vi "SetBuildVersionCaller.vi"(11 "Command line arguments \nfor the VI":string[](array[string])) -> (2 "Output or error information to include in \nthe CLI for LabVIEW console or log file.":string, 3 "CLI for LabVIEW exit code that the VI returns":i32)   [LabVIEW 2020]
doc: "Calls SetBuildVersion.vi to set the version of the build specification."
uses:
  <vilib>/AppBuilder/AB_API_Simple/Build Specification Version.ctl
  <vilib>/AppBuilder/AB_API_Simple/NI_App_Builder_API.lvlib
panel:
  out "error out":errorcluster
  in  "error in (no error)":errorcluster
  out "Set Version":T1
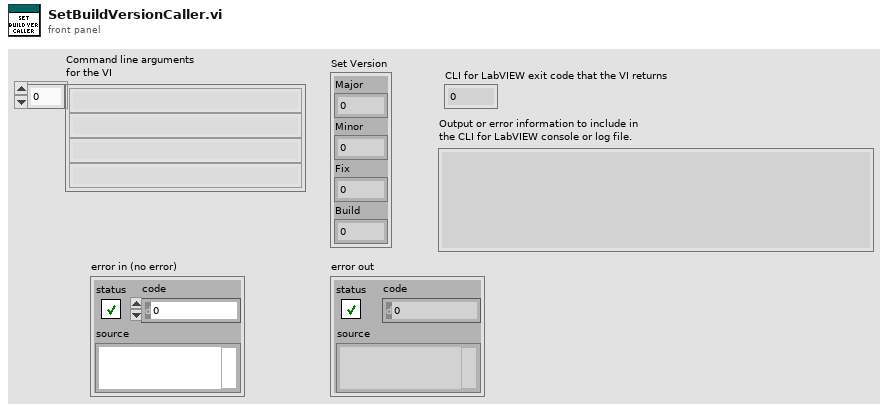
[diagram p1: front panel]
types:
  T1 = typedef "NI_App_Builder_API.lvlib/Build Specification Version.ctl" = cluster{"Major":u16, "Minor":u16, "Fix":u16, "Build":u16}
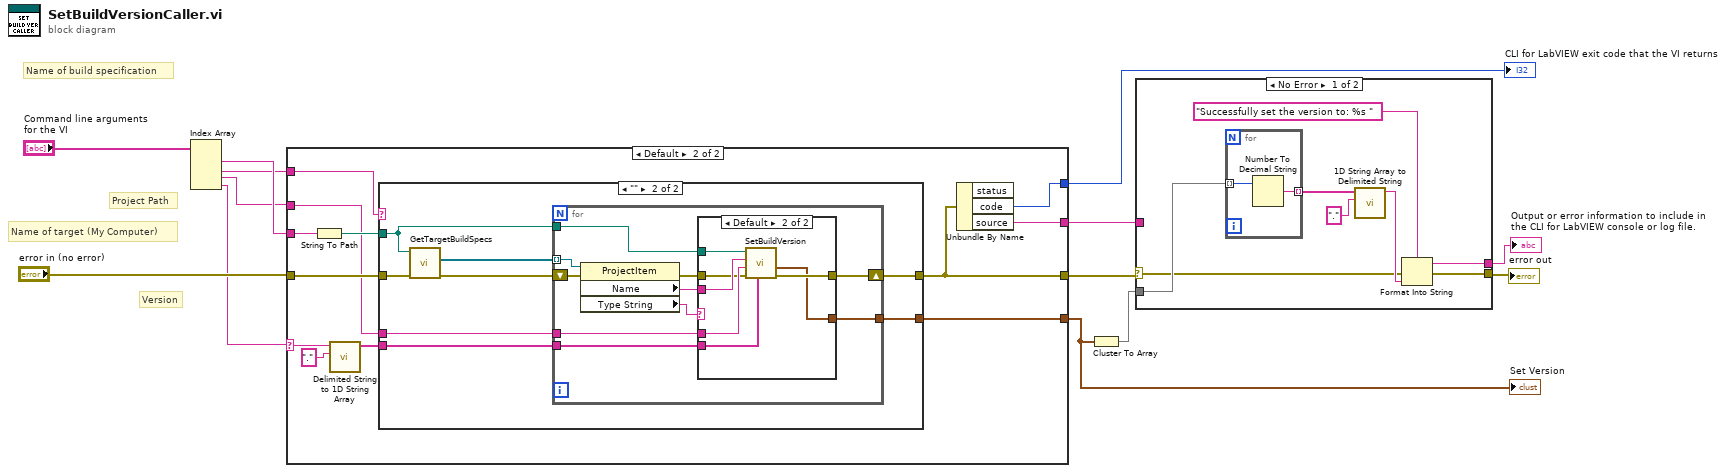
[diagram p0: block diagram]
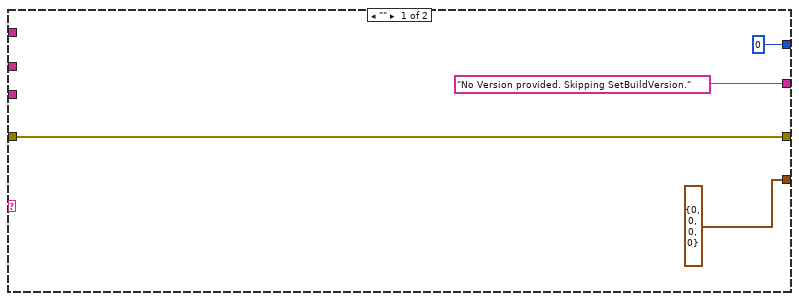
[diagram p3: hidden frame]
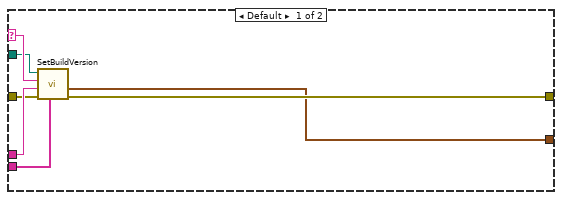
[diagram p4: hidden frame]
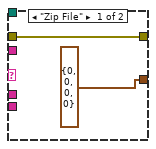
[diagram p5: hidden frame]
diagram:
  # "Project Path"
  # "Version"
  # "Name of target (My Computer)"
  # "Name of build specification"
  n1 = Index Array(array="Command line arguments \nfor the VI") -> (element #1=w11:string, element #2=w8:string, element #3=w9:string, element #4=w7:string)  [unwired: 4 in]
  n2 = case shown="Default" w7 {
    selector: w7 -> [_ w24]
    tunnel: [T1 {"Major"=0, "Minor"=0, "Fix"=0, "Build"=0} ("Set Version") w20] -> w4
    tunnel: ["No Version provided. Skipping SetBuildVersion." ("source") w28] -> w1
    tunnel: [0 ("code") w27] -> w13
    tunnel: [w17 w21] -> w6
    tunnel: w11 -> [_ w26]
    tunnel: "error in (no error)" -> [w17 w22]
    tunnel: w9 -> [_ w19]
    tunnel: w8 -> [_ w25]
    frame "" {
    }
    frame Default {
      n3 = String To Path(string=w26) -> (path=w23:path)
      n4 = call <vilib>:"Delimited String to 1D String Array.vi"("delimiter"=".", "delimited string"=w24) -> ("string array"=w18:string[])  [unwired: 9 in]
      n5 = case shown="\"\"" w25 {
        selector: w25 -> [w36 _]
        tunnel: w23 -> [w30 w37]
        tunnel: w22 -> [w33 w43]
        tunnel: [w32 w41] -> w21
        tunnel: [w31 w40] -> w20
        tunnel: w19 -> [w35 w39]
        tunnel: w18 -> [w34 w38]
        frame Default {
          n6 = call "SetBuildVersion.vi"("Version (delimited)"=w34, "error in (no error)"=w33, "Target Name"=w35, "Name of build specification"=w36, "Path to project"=w30) -> ("error out"=w32:errorcluster, "Set Version"=w31:T1)  [unwired: 5 in]
        }
        frame "" {
          n7 = call <vilib>:"GetTargetBuildSpecs.vi"("error in (no error)"=w43, "Path to project"=w37) -> ("error out"=w42:errorcluster, "buildspec refs"=w44:refnum<vi>[])  [unwired: 2 in, 6 out]
          n8 = for {
            tunnel: w44 -> [w54] mode=indexing
            shift-right: [w53] -> w41
            shift-left: w42 -> [w47]
            tunnel: [w52] -> w40
            tunnel: w39 -> [w51]
            tunnel: w38 -> [w50]
            tunnel: w37 -> [w48]
            n9 = property on="Property Node" class="ProjectItem"(reference=w54, error in=w47) -> (error out=w46:errorcluster, "Name"=w49:string, "Type String"=w45:string)  [unwired: 1 out]
            n10 = case shown="Default" w45 {
              tunnel: [w56 w63] -> w53
              tunnel: [T1 {"Major"=0, "Minor"=0, "Fix"=0, "Build"=0} ("Set Version") w62] -> w52
              tunnel: w51 -> [_ w61]
              tunnel: w50 -> [_ w60]
              tunnel: w49 -> [_ w59]
              tunnel: w48 -> [_ w58]
              tunnel: w46 -> [w56 w57]
              frame "Zip File" {
              }
              frame Default {
                n11 = call "SetBuildVersion.vi"("Version (delimited)"=w60, "error in (no error)"=w57, "Target Name"=w61, "Name of build specification"=w59, "Path to project"=w58) -> ("error out"=w63:errorcluster, "Set Version"=w62:T1)  [unwired: 5 in]
              }
            }
          }
        }
      }
      n12 = Unbundle By Name(w21) -> ("code"=w27:i32, "source"=w28:string)  [unwired: 1 out]
    }
  }
  "Set Version" <- w4
  "CLI for LabVIEW exit code that the VI returns" <- w13
  n13 = Cluster To Array(cluster=w4) -> (array=w3:u16[])
  n14 = case shown="No Error" w6 {
    selector: w6 -> [w65 w75]
    tunnel: [w66 w75] -> w5
    tunnel: w3 -> [w68 _]
    tunnel: [w64 w74] -> w2
    tunnel: w1 -> [_ w74]
    frame No Error {
      n15 = for {
        tunnel: w68 -> [w73] mode=indexing
        tunnel: [w72] -> w70 mode=indexing
        n16 = Number To Decimal String(number=w73) -> (decimal integer string=w72:string)  [unwired: 1 in]
      }
      n17 = call <vilib>:"1D String Array to Delimited String.vi"("delimiter"=".", "string array"=w70) -> ("delimited string"=w71:string)  [unwired: 9 in]
      n18 = Format Into String(format string="Successfully set the version to: %s " ("Text to Write"), error in=w65, w71) -> (resulting string=w64:string, error out=w66:errorcluster)  [unwired: 1 in]
    }
    frame Error {
    }
  }
  "error out" <- w5
  "Output or error information to include in \nthe CLI for LabVIEW console or log file." <- w2
